vi "Translate_LISTBOX.vi"(8 "error IN":errorcluster, 10 "Cle":string, 11 "LstBox Refnum":refnum<vi>) -> (0 "error out":errorcluster)   [LabVIEW 2013]
uses:
  Dictionnary/EnumCommandDictionnaire.ctl
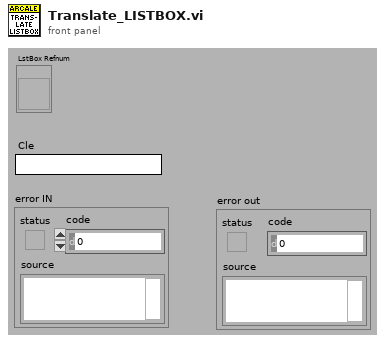
[diagram p1: front panel]
types:
  T1 = typedef "EnumCommandDictionnaire.ctl" = enum16{"Load", "Translate", "Save", "GetDico", "Set : A traduire = Vrai", "Set : A Traduire = Faux", "SetDico"}
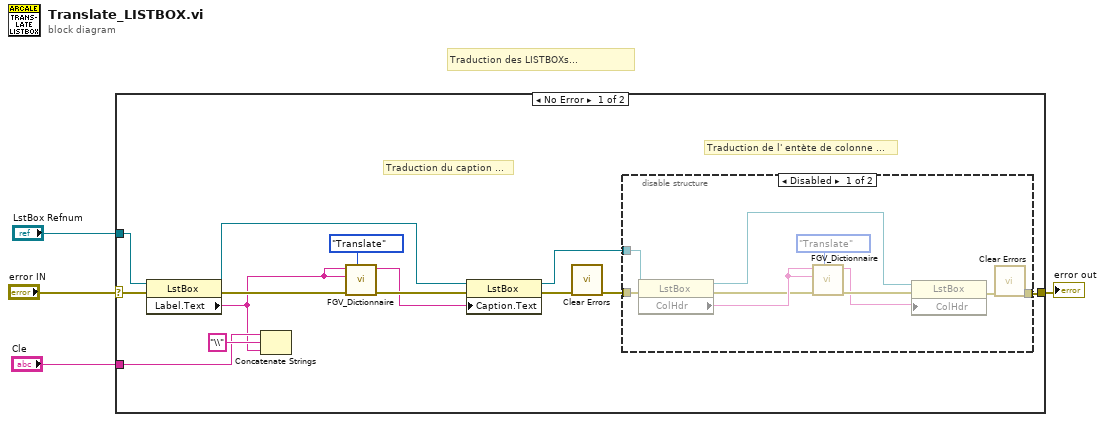
[diagram p0: block diagram]
diagram:
  # "Traduction des LISTBOXs..."
  n1 = case shown="No Error" "error IN" {
    selector: "error IN" -> [w18 w30]
    tunnel: "LstBox Refnum" -> [w17 _]
    tunnel: "Cle" -> [w13 _]
    tunnel: [w5 w30] -> w1
    frame No Error {
      # "Traduction de l' entète de colonne ..."
      # "Traduction du caption ..."
      n2 = property class="LstBox"(reference=w17, error in=w18) -> (reference out=w14:refnum<vi>, error out=w11:errorcluster, "Label.Text"=w8:string)
      n3 = Concatenate Strings(w13, "\\" ("string"), w8) -> ()  [unwired: 1 out]
      n4 = call "FGV_Dictionnaire.vi"("Command"=EnumCommandDictionnaire."Translate", "error in (no error)"=w11, "Chaîne"=w8, "Clé"=w8) -> ("error out"=w10:errorcluster, "Traduction"=w9:string)  [unwired: 5 in, 1 out]
      n5 = property class="LstBox"(reference=w14, error in=w10, "Caption.Text"=w9) -> (reference out=w6:refnum<vi>, error out=w15:errorcluster)
      n6 = call <vilib>:"Clear Errors.vi"("error in (no error)"=w15) -> ("error out"=w7:errorcluster)  [unwired: 6 in]
      n7 = disable-structure shown="Disabled" {
        disable-tunnel: w7 -> [w28 w29]
        disable-tunnel: w6 -> [w27 _]
        disable-tunnel: [w22 w29] -> w5
        frame Disabled {
          n8 = property class="LstBox"(reference=w27, error in=w28) -> (reference out=w20:refnum<vi>, error out=w25:errorcluster, "ColHdr"=w26:string)
          n9 = call "FGV_Dictionnaire.vi"("Command"=EnumCommandDictionnaire."Translate", "error in (no error)"=w25, "Chaîne"=w26, "Clé"=w26) -> ("error out"=w24:errorcluster, "Traduction"=w21:string)  [unwired: 5 in, 1 out]
          n10 = property class="LstBox"(reference=w20, error in=w24, "ColHdr"=w21) -> (error out=w23:errorcluster)  [unwired: 1 out]
          n11 = call <vilib>:"Clear Errors.vi"("error in (no error)"=w23) -> ("error out"=w22:errorcluster)  [unwired: 6 in]
        }
        frame Enabled {
        }
      }
    }
    frame Error {
    }
  }
  "error out" <- w1
